vi "Basic Function Test.vi"() -> (0 "error out":errorcluster)   [LabVIEW 2014, in "SQLite3LV Tests.lvlib"]
uses:
  SQLite3LV Tests.lvlib
  SQLite3LV/Cursor Class/property binding/column count.vi
  SQLite3LV/SQLite3 Class/sqlite3.lvclass
  SQLite3LV/Cursor Class/cursor.lvclass
panel:
  out "Column Count?":i32
  out "Array":string[][](array[string])
  in  "statement":string="CREATE TABLE Persons\n(\nID int PRIMARY KEY,\nLastName varchar(255),\nFirstName varchar(255)\n);\nINSERT INTO Persons VALUES\n(0, \"Doe\", \"John\");\nINSERT INTO Persons VALUES\n(1, \"White\", \"Sarah\");\nINSERT INTO Persons VALUES\n(2, \"Bacon\", \"Kevin\");\nSELECT * FROM Persons;"
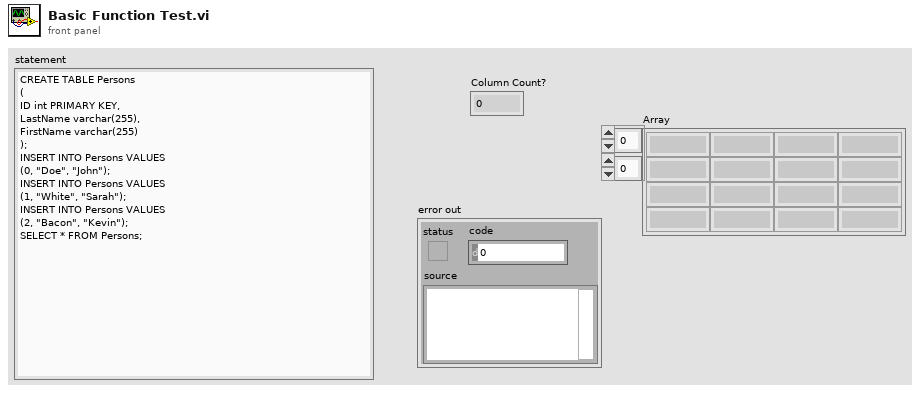
[diagram p1: front panel]
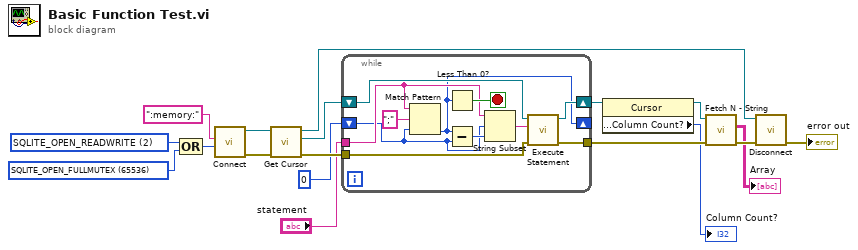
[diagram p0: block diagram]
diagram:
  w17 = u32 65536 items=["SQLITE_OPEN_READONLY"=1, "SQLITE_OPEN_READWRITE"=2, "SQLITE_OPEN_CREATE"=4, "SQLITE_OPEN_DELETEONCLOSE"=8, "SQLITE_OPEN_EXCLUSIVE"=16, "SQLITE_OPEN_AUTOPROXY"=32, "SQLITE_OPEN_URI"=64, "SQLITE_OPEN_MEMORY"=128, "SQLITE_OPEN_MAIN_DB"=256, "SQLITE_OPEN_TEMP_DB"=512, "SQLITE_OPEN_TRANSIENT_DB"=1024, "SQLITE_OPEN_MAIN_JOURNAL"=2048, "SQLITE_OPEN_TEMP_JOURNAL"=4096, "SQLITE_OPEN_SUBJOURNAL"=8192, "SQLITE_OPEN_MASTER_JOURNAL"=16384, "SQLITE_OPEN_NOMUTEX"=32768, "SQLITE_OPEN_FULLMUTEX"=65536, "SQLITE_OPEN_SHAREDCACHE"=131072, "SQLITE_OPEN_PRIVATECACHE"=262144, "SQLITE_OPEN_WAL"=524288] ("SQLITE3 Open Flag")
  w18 = u32 2 items=["SQLITE_OPEN_READONLY"=1, "SQLITE_OPEN_READWRITE"=2, "SQLITE_OPEN_CREATE"=4, "SQLITE_OPEN_DELETEONCLOSE"=8, "SQLITE_OPEN_EXCLUSIVE"=16, "SQLITE_OPEN_AUTOPROXY"=32, "SQLITE_OPEN_URI"=64, "SQLITE_OPEN_MEMORY"=128, "SQLITE_OPEN_MAIN_DB"=256, "SQLITE_OPEN_TEMP_DB"=512, "SQLITE_OPEN_TRANSIENT_DB"=1024, "SQLITE_OPEN_MAIN_JOURNAL"=2048, "SQLITE_OPEN_TEMP_JOURNAL"=4096, "SQLITE_OPEN_SUBJOURNAL"=8192, "SQLITE_OPEN_MASTER_JOURNAL"=16384, "SQLITE_OPEN_NOMUTEX"=32768, "SQLITE_OPEN_FULLMUTEX"=65536, "SQLITE_OPEN_SHAREDCACHE"=131072, "SQLITE_OPEN_PRIVATECACHE"=262144, "SQLITE_OPEN_WAL"=524288] ("SQLITE3 Open Flag")
  n1 = Compound Arithmetic op=OR(w18, w17) -> (w15:u32)
  n2 = call "Connect.vi"("SQLITE3 open flags"=w15, "path"=":memory:" ("path_utf8")) -> ("error out"=w13:errorcluster, "SQLite3LV Connection out"=w14:refnum<class "sqlite3.lvclass">)  [unwired: 8 in]
  n3 = call "Get Cursor.vi"("error in (no error)"=w13, "SQLite3LV Connection in"=w14) -> ("error out"=w9:errorcluster, "SQLite3LV Cursor"=w12:refnum<class "cursor.lvclass">, "SQLite3LV Connection out"=w7:refnum<class "sqlite3.lvclass">)  [unwired: 7 in]
  n4 = while {
    tunnel: [w27] -> w10
    tunnel: w9 -> [w26]
    shift-right: [w20] -> _
    shift-left: 0 -> [w19]
    tunnel: "statement" -> [w22]
    shift-right: [w28] -> w11
    shift-left: w12 -> [w29]
    stop <- w25 stop-if-true
    n5 = Match Pattern(string=w22, regular expression=";", offset (0)=w19) -> (offset past match=w20:i32)  [unwired: 3 out]
    n6 = Less Than 0?(x=w20) -> (x < 0?=w25:bool)
    n7 = Subtract(x=w20, y=w19) -> (x-y=w24:i32)
    n8 = String Subset(string=w22, offset (0)=w19, length (rest)=w24) -> (substring=w23:string)
    n9 = call "Execute Statement.vi"("error in (no error)"=w26, "SQL statement"=w23, "SQLite3LV Cursor in"=w29) -> ("error out"=w27:errorcluster, "SQLite3LV Cursor out"=w28:refnum<class "cursor.lvclass">)  [unwired: 7 in]
  }
  n10 = property class="Cursor"(reference=w11) -> (reference out=w2:refnum<class "cursor.lvclass">, "property binding:Column Count?"=→"Column Count?":i32)  [unwired: 1 in, 1 out]
  n11 = call "Fetch N - String.vi"("error in (no error)"=w10, "SQLite3LV Cursor in"=w2) -> ("error out"=w8:errorcluster, "result"=→"Array":string[][])  [unwired: 6 in, 2 out]
  n12 = call "Disconnect.vi"("error in (no error)"=w8, "SQLite3LV Connection in"=w7) -> ("error out"=→"error out":errorcluster)  [unwired: 9 in]
